vi "Actor Core.vi"(8 "error in":errorcluster, 11 "DIMActor in":refnum<class "DIMActor.lvclass">) -> (0 "error out":errorcluster, 3 "Actor out":refnum<class "Actor.lvclass">)   [LabVIEW 2012, in "DIMActor.lvlib" / "DIMActor.lvclass"]
doc: "(<B>Filename</B>: Actor Framework.lvlib:Actor.lvclass:Actor Core.vi)\n\nReceives messages to the actor, reacts to them, and initiates any error handling that may shut the actor down.\n\nDescendant classes may override this VI to append parallel tasks for the actor to complete while it handles messages. Overrides use the Call Parent Method node."
uses:
  DIMActor.lvclass
  <vilib>/ActorFramework/Actor/Actor.lvclass
  DIMActor.lvclass/DIMActor.ctl
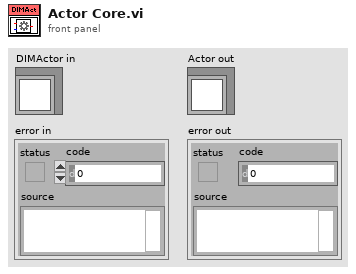
[diagram p1: front panel]
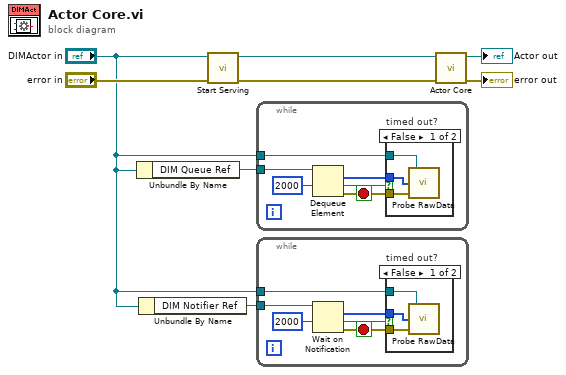
[diagram p0: block diagram]
diagram:
  n1 = Unbundle By Name("DIMActor in") -> ("DIM Queue Ref"=w1:refnum<queue>)
  n2 = Unbundle By Name("DIMActor in") -> ("DIM Notifier Ref"=w3:refnum<notifier>)
  n3 = call "Start Serving.vi"("error in (no error)"="error in", "DIMActor in"="DIMActor in") -> ("error out"=w5:errorcluster, "DIMActor out"=w6:refnum<class "DIMActor.lvclass">)  [unwired: 8 in]
  n4 = while {
    tunnel: w1 -> [w14]
    tunnel: "DIMActor in" -> [w10]
    stop <- w12 stop-if-true
    n5 = Dequeue Element(queue=w14, timeout in ms (-1)=2000) -> (element=w9:i8[], timed out?=w11:bool, error out=w12:errorcluster)  [unwired: 1 in, 1 out]
    n6 = case "timed out?" shown="False" w11 {
      tunnel: w9 -> [w17 _]
      tunnel: w12 -> [w16 _]
      tunnel: w10 -> [w15 _]
      frame False {
        n7 = call "Probe RawData.vi"("Error In"=w16, "Raw Data"=w17, "DIMActor"=w15) -> ()  [unwired: 2 in, 1 out]
      }
      frame True {
      }
    }
  }
  n8 = while {
    tunnel: w3 -> [w23]
    tunnel: "DIMActor in" -> [w18]
    stop <- w21 stop-if-true
    n9 = Wait on Notification(notifier=w23, timeout in ms (-1)=2000) -> (notification=w19:i8[], timed out?=w20:bool, error out=w21:errorcluster)  [unwired: 2 in, 1 out]
    n10 = case "timed out?" shown="False" w20 {
      tunnel: w19 -> [w26 _]
      tunnel: w21 -> [w25 _]
      tunnel: w18 -> [w24 _]
      frame False {
        n11 = call "Probe RawData.vi"("Error In"=w25, "Raw Data"=w26, "DIMActor"=w24) -> ()  [unwired: 2 in, 1 out]
      }
      frame True {
      }
    }
  }
  n12 = call-parent "Actor Core.vi"("error in"=w5, "Actor in"=w6) -> ("error out"=→"error out":errorcluster, "Actor out"=→"Actor out":refnum<class "Actor.lvclass">)  [unwired: 8 in]
